vi "Main.vi"() -> ()   [LabVIEW 2013]
uses:
  Ctl/States.ctl
  Ctl/Setup.ctl
  GlobValue.vi
panel:
  out "SN_Head":string
  out "SN_Length":i32
  out "error out":errorcluster caption="错误输出"
  in  "IdentifyReady":bool
  in  "SlotReady":bool
  out "直通率":string
  out "Failed":u32
  out "Tested":u32
  out "Passed":u32
  in  "Next":bool
  out "测试失败项目":string
  in  "Starttime":u32
  out "Pass Yeild":dbl(graph)
  in  "GUIRef":T1
  in  "Start":bool
  in  "测试模式":u16(ring) items=["生产模式", "调试模式", "循环模式", "停止测试"]
  in  "循环次数":u32
  in  "产品标识":string
  out "测试结果":bool
  out "TBOX状态":bool
  in  "CheckOut":bool
  in  "Clear":bool
  out "进度条":i32(slide) scale=0.0..100.0
  out "测试时间":dbl
  out "分类测试结果":T2
  in  "中止":bool
  in  "Setup":bool
  out "运行Log":string
  in  "测试结果栏":i32(listbox)
  out "测试状态":string
  in  "Return":bool
  in  "产品名称":string
  in  "产品型号":u16(ring) items=["1802", "1805", "1831"]
  # "休眠唤醒测试"
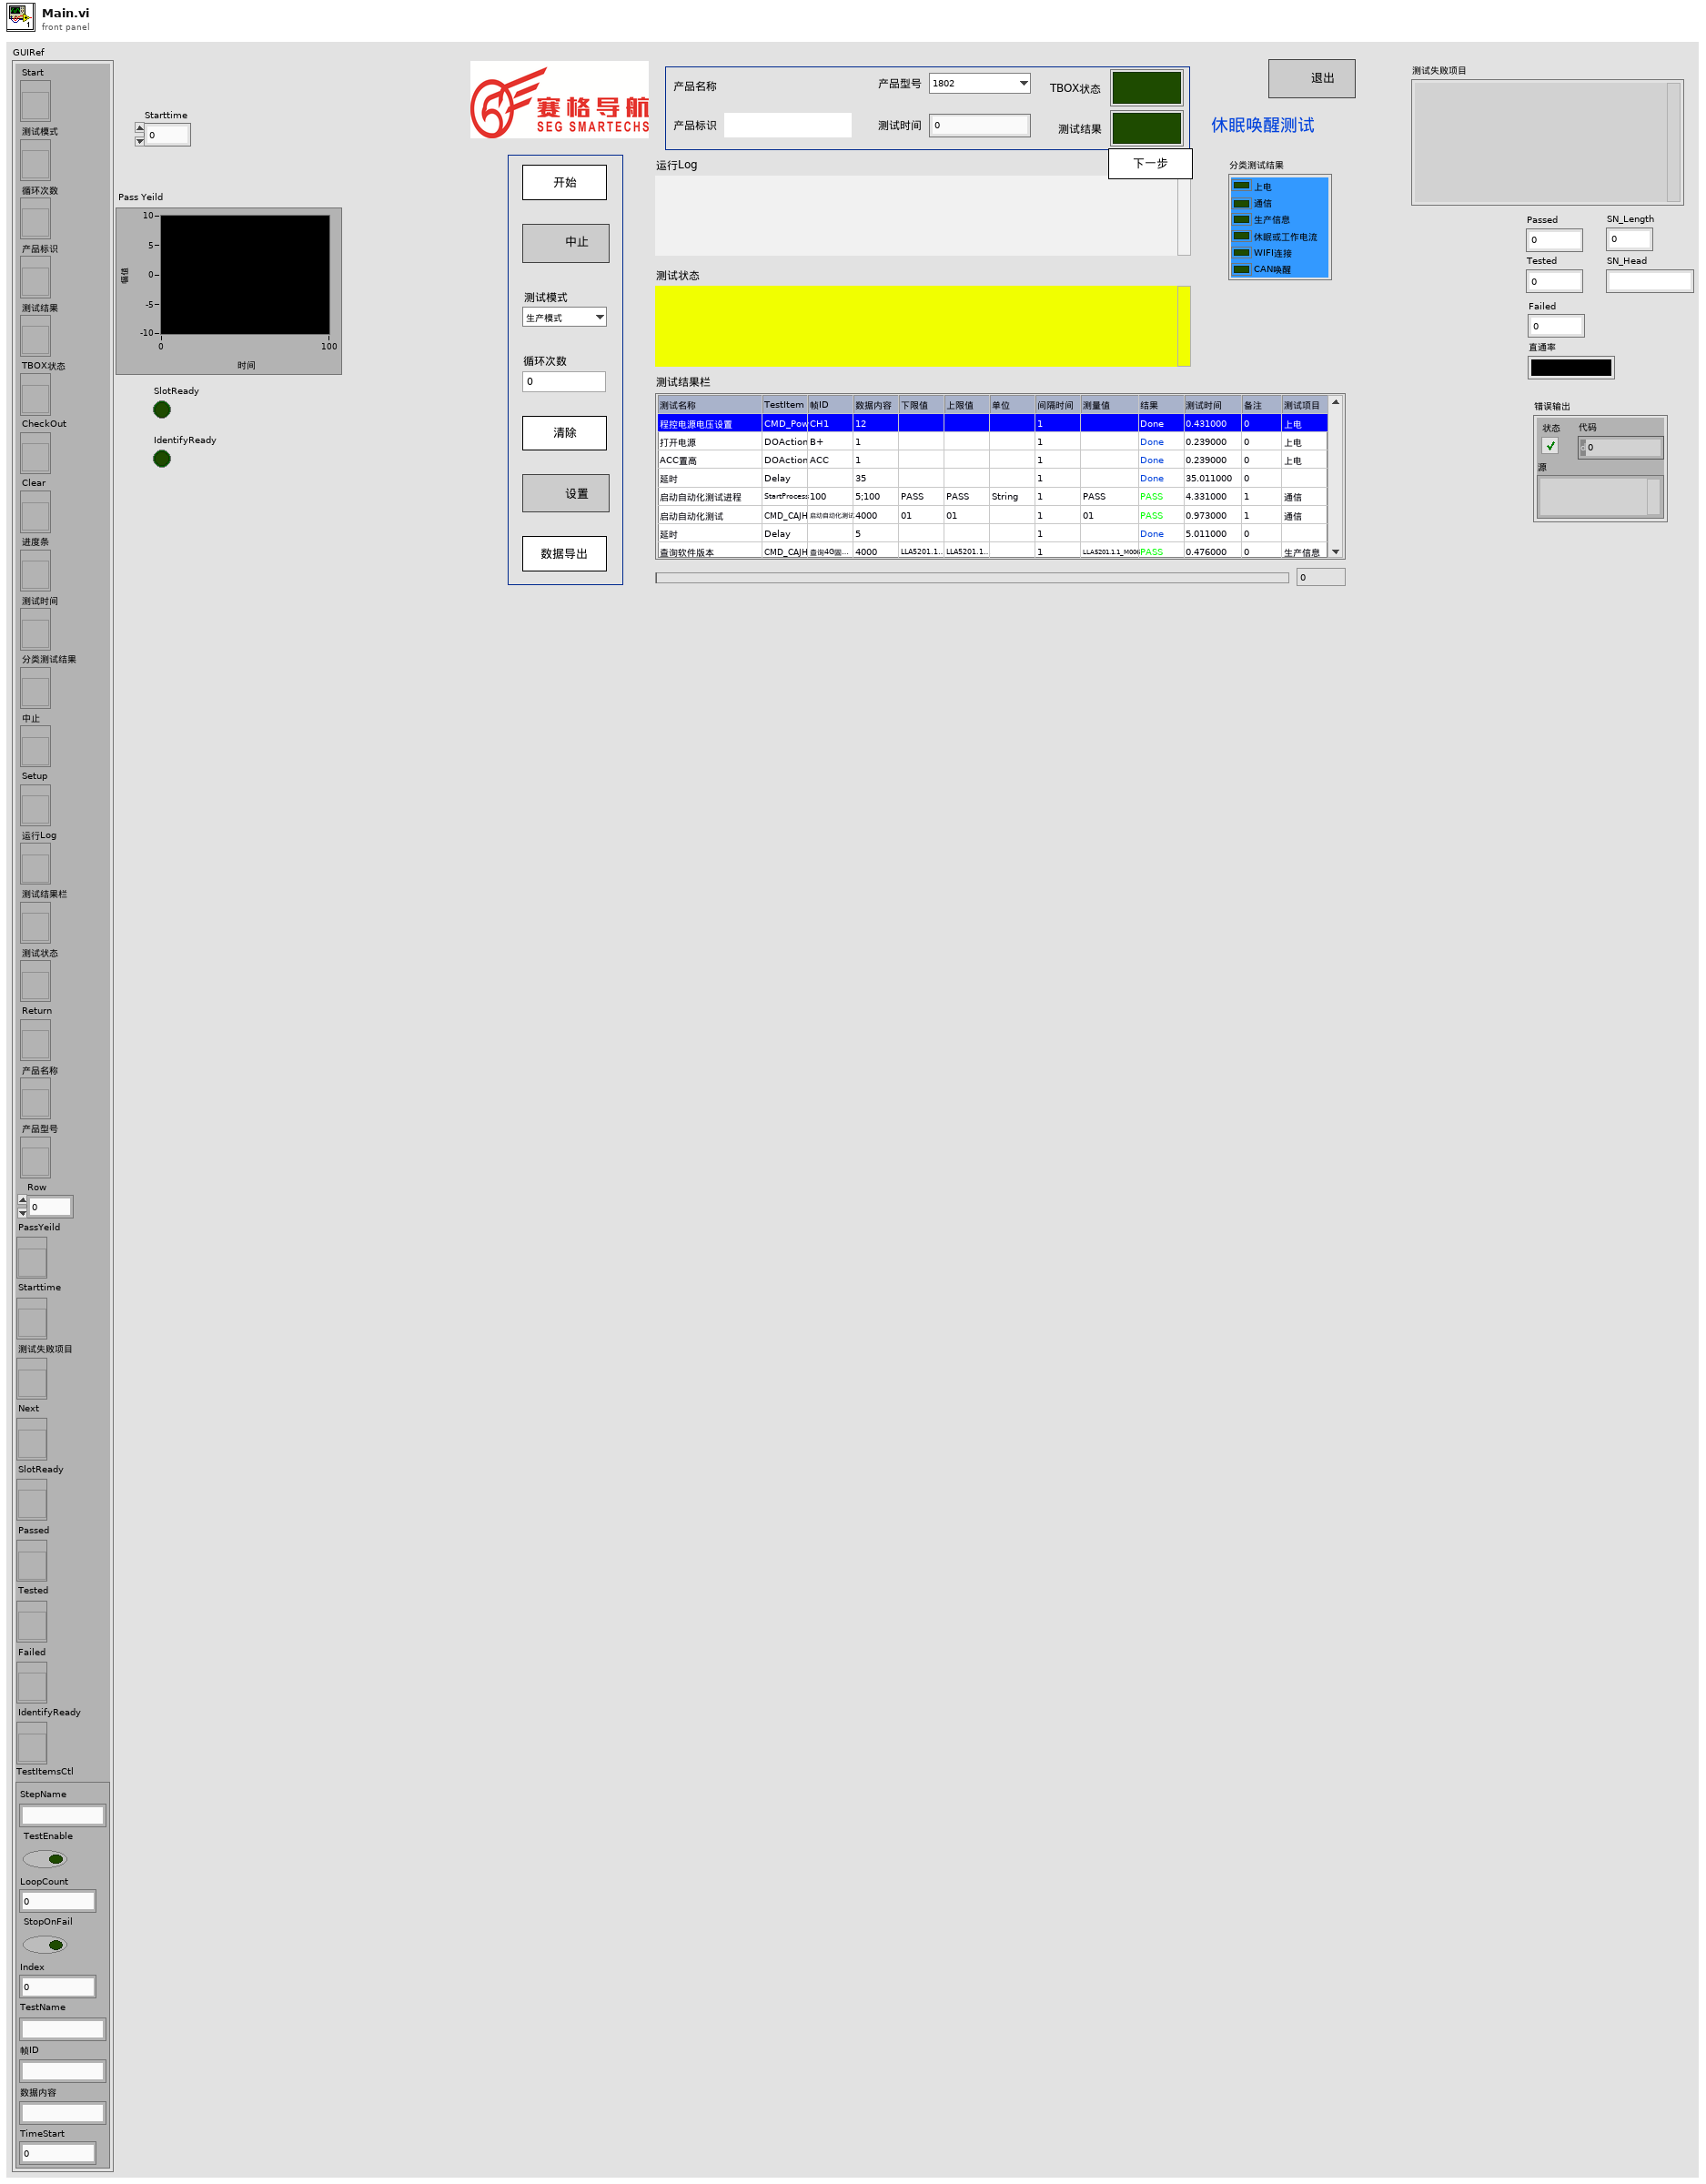
[diagram p1: front panel]
types:
  T1 = typedef "控件.ctl" = cluster{"Start":refnum<vi>, "测试模式":refnum<vi>, "循环次数":refnum<vi>, "产品标识":refnum<vi>, "测试结果":refnum<vi>, "TBOX状态":refnum<vi>, "CheckOut":refnum<vi>, "Clear":refnum<vi>, "进度条":refnum<vi>, "测试时间":refnum<vi>, "分类测试结果":refnum<vi>, "中止":refnum<vi>, "Setup":refnum<vi>, "运行Log":refnum<vi>, "测试结果栏":refnum<vi>, "测试状态":refnum<vi>, "Return":refnum<vi>, "产品名称":refnum<vi>, "产品型号":refnum<vi>, "Row":i32, "PassYeild":refnum<vi>, "Starttime":refnum<vi>, "测试失败项目":refnum<vi>, "Next":refnum<vi>, "SlotReady":refnum<vi>, "Passed":refnum<vi>, "Tested":refnum<vi>, "Failed":refnum<vi>, "IdentifyReady":refnum<vi>, "TestItemsCtl":cluster{"StepName":string, "TestEnable":bool, "LoopCount":u32, "StopOnFail":bool, "Index":u32, "TestName":string, "帧ID":string, "数据内容":string, "TimeStart":u32}}
  T2 = cluster{"电流":bool, "SD卡":bool, "USB":bool, "收音机":bool, "DVD":bool, "蓝牙":bool, "IPOD":bool, "终端":bool, "数字电视":bool, "AuxIn":bool, "按键":bool, "ILL检测":bool, "刹车检测":bool, "倒车检测":bool, "方控":bool, "导航":bool, "USB1":bool}
  T3 = enum8{"Enabled", "Disabled", "Disabled and Grayed Out"}
  T4 = typedef "States.ctl" = enum16{"Init", "PreUUT", "Idle", "SetUp", "TestSequence", "PostUUT", "StopTest", "Debug Mode", "Selection Mode", "Loop Mode", "Error", "Wait"}
  T5 = typedef "Setup.ctl" = cluster{"TestedNum":u32, "PassedNum":u32, "FailedNum":u32, "Slot1TestedNum":u32, "Slot2TestedNum":u32, "Slot3TestedNum":u32, "Slot4TestedNum":u32, "GuiVer":string, "LimitFileVer":string, "Login Name":string, "Password":string, "SN_Head":string, "SN_Length":i32, "AbortOnFail":bool, "DataBaseEnable?":bool, "FixtureID":string, "ShowSkipStep?":bool}
  T6 = enum32{"invalid app kind", "Development System", "Run Time System", "Student Edition", "Embedded LabVIEW", "Evaluation", "Custom"}
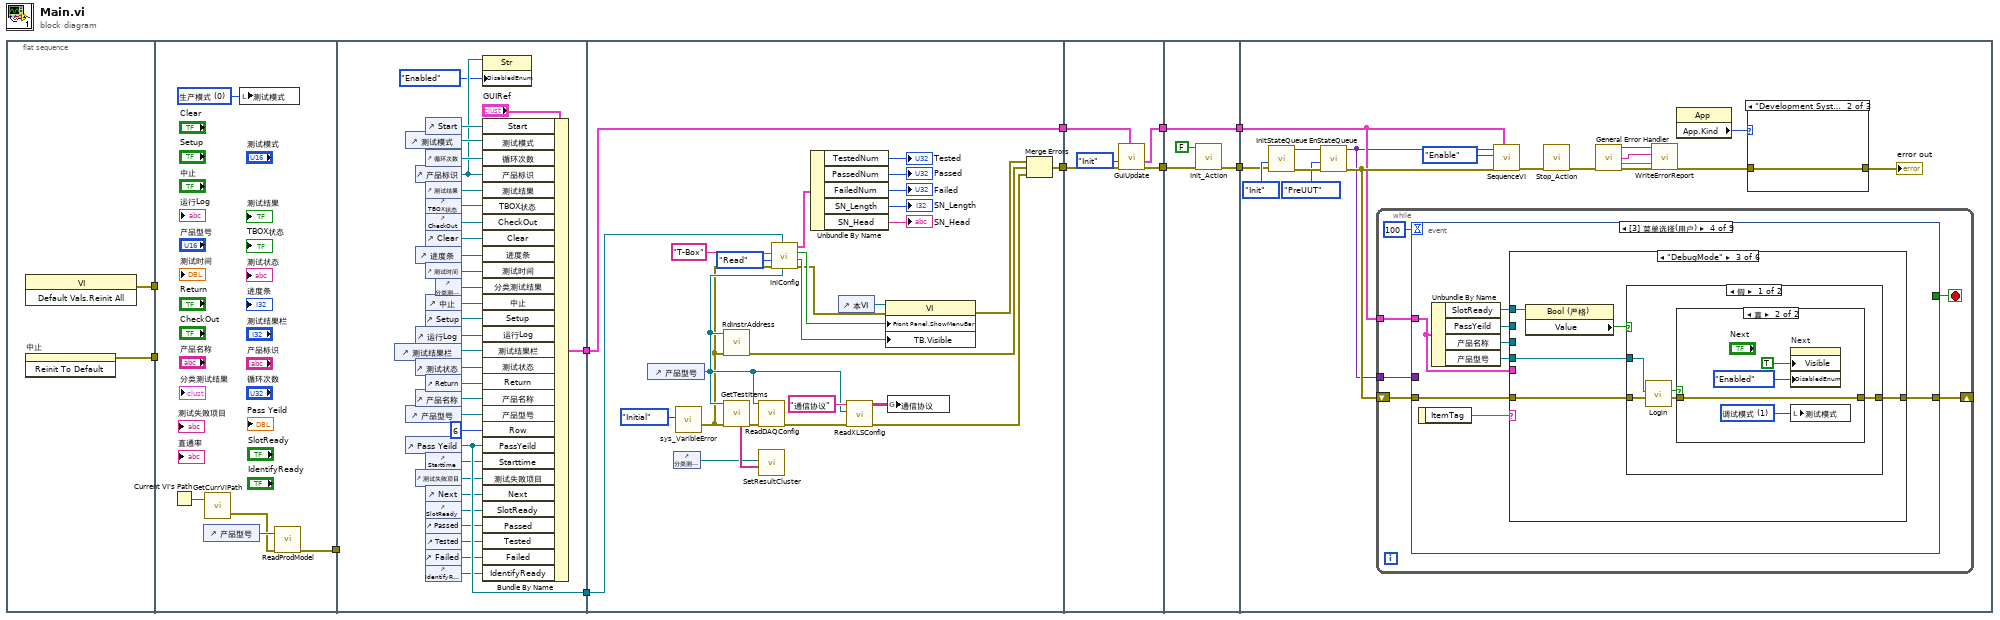
[diagram p0: block diagram]
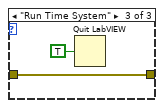
[diagram p3: hidden frame]
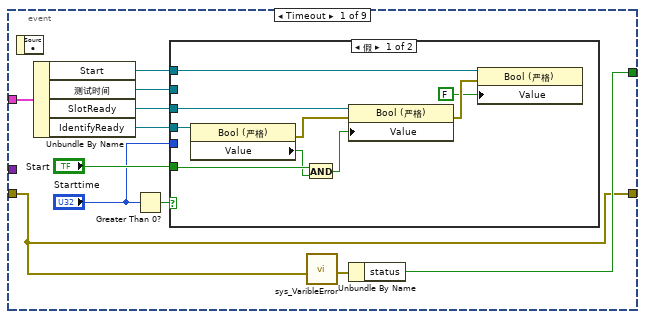
[diagram p4: hidden frame]
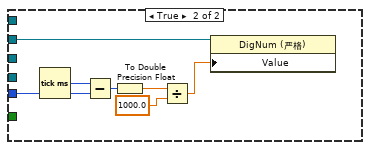
[diagram p5: hidden frame]
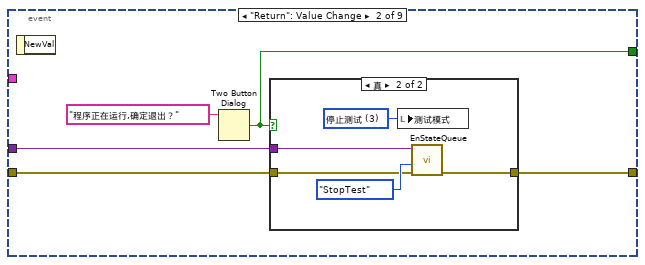
[diagram p6: hidden frame]
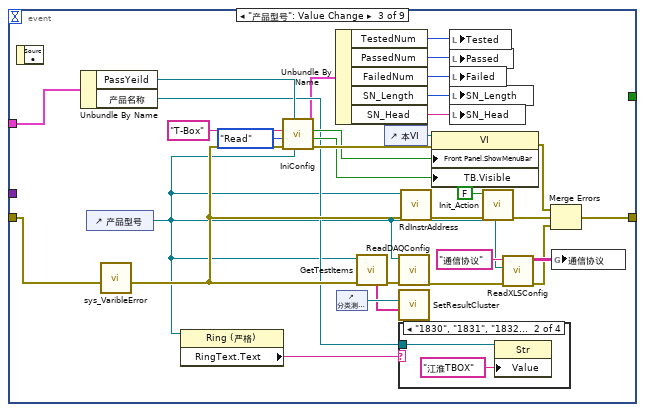
[diagram p8: hidden frame]
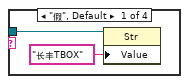
[diagram p9: hidden frame]
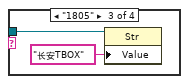
[diagram p10: hidden frame]
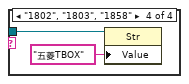
[diagram p11: hidden frame]
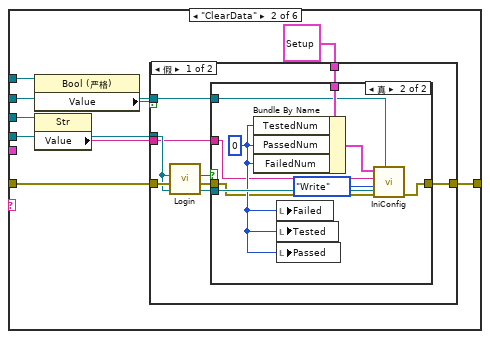
[diagram p13: hidden frame]
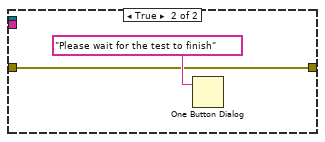
[diagram p15: hidden frame]
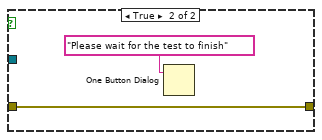
[diagram p17: hidden frame]
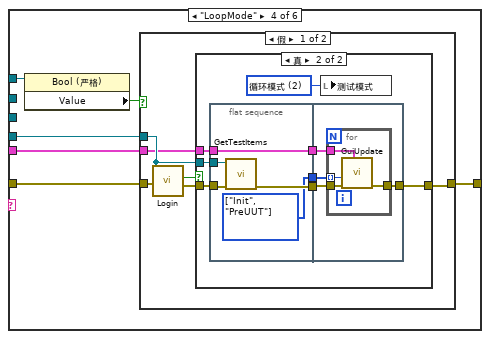
[diagram p18: hidden frame]
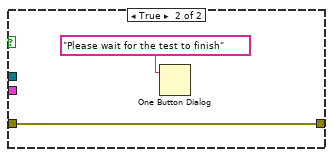
[diagram p20: hidden frame]
diagram:
  n1 = flat-sequence {
    tunnel: [w13] -> w11
    tunnel: [w12] -> w1
    tunnel: w11 -> [_]
    tunnel: [w15] -> w5
    tunnel: w1 -> [_]
    tunnel: [w31] -> w10
    tunnel: [w30] -> w9
    tunnel: w5 -> [_]
    tunnel: w10 -> [w57]
    tunnel: w9 -> [w63]
    tunnel: [w58] -> w8
    tunnel: [w57] -> w7
    tunnel: w8 -> [w82]
    tunnel: w7 -> [w79]
    tunnel: [w80] -> w6
    tunnel: [w78] -> w2
    tunnel: w6 -> [w86]
    tunnel: [w85] -> w4
    tunnel: [w84] -> w3
    tunnel: w2 -> [w84]
    tunnel: w4 -> [w102]
    tunnel: w3 -> [w88]
    frame #0 {
      n2 = invoke class="VI" method="Default Vals.Reinit All"() -> (error out=w13:errorcluster)  [unwired: 3 in, 2 out]
      n3 = invoke on="中止" class="Bool (严格)" method="Reinit To Default"() -> (error out=w12:errorcluster)  [unwired: 3 in, 2 out]
    }
    frame #1 {
      w17 = u16 0 items=["生产模式", "调试模式", "循环模式", "停止测试"] ("测试模式")
      n4 = Current VI's Path() -> (path=w18:path)
      n5 = control-ref of="产品型号"() -> (w16:refnum<vi>)
      n6 = call "GetCurrViPath.vi"("PathIn"=w18) -> ("error out"=w14:errorcluster)  [unwired: 1 in, 1 out]
      n7 = local write "测试模式"(w17) -> ()
      n8 = call "ReadProdModel.vi"("error in"=w14, "产品型号"=w16) -> ("error out"=w15:errorcluster)  [unwired: 9 in]
    }
    frame #2 {
      n9 = control-ref of="测试结果栏"() -> (w37:refnum<vi>)
      n10 = control-ref of="测试模式"() -> (w48:refnum<vi>)
      n11 = control-ref of="产品型号"() -> (w33:refnum<vi>)
      n12 = control-ref of="Pass Yeild"() -> (w30:refnum<vi>)
      n13 = control-ref of="产品标识"() -> (w20:refnum<vi>)
      n14 = control-ref of="进度条"() -> (w43:refnum<vi>)
      n15 = control-ref of="运行Log"() -> (w38:refnum<vi>)
      n16 = control-ref of="测试状态"() -> (w36:refnum<vi>)
      n17 = control-ref of="产品名称"() -> (w34:refnum<vi>)
      n18 = control-ref of="测试失败项目"() -> (w28:refnum<vi>)
      n19 = control-ref of="Start"() -> (w49:refnum<vi>)
      n20 = control-ref of="循环次数"() -> (w27:refnum<vi>)
      n21 = control-ref of="测试结果"() -> (w47:refnum<vi>)
      n22 = control-ref of="TBOX状态"() -> (w46:refnum<vi>)
      n23 = control-ref of="CheckOut"() -> (w45:refnum<vi>)
      n24 = control-ref of="Clear"() -> (w44:refnum<vi>)
      n25 = control-ref of="测试时间"() -> (w42:refnum<vi>)
      n26 = control-ref of="中止"() -> (w40:refnum<vi>)
      n27 = control-ref of="Setup"() -> (w39:refnum<vi>)
      n28 = control-ref of="Return"() -> (w35:refnum<vi>)
      n29 = control-ref of="Starttime"() -> (w29:refnum<vi>)
      n30 = control-ref of="Next"() -> (w25:refnum<vi>)
      n31 = control-ref of="SlotReady"() -> (w26:refnum<vi>)
      n32 = control-ref of="Passed"() -> (w24:refnum<vi>)
      n33 = control-ref of="Tested"() -> (w23:refnum<vi>)
      n34 = control-ref of="Failed"() -> (w22:refnum<vi>)
      n35 = control-ref of="IdentifyReady"() -> (w21:refnum<vi>)
      n36 = control-ref of="分类测试结果"() -> (w41:refnum<vi>)
      n37 = property class="Str"(reference=w20, "DisabledEnum"=T3."Enabled" ("禁用")) -> ()  [unwired: 1 in, 2 out]
      n38 = Bundle By Name(cluster="GUIRef", "Start"=w49, "测试模式"=w48, "循环次数"=w27, "产品标识"=w20, "测试结果"=w47, "TBOX状态"=w46, "CheckOut"=w45, "Clear"=w44, "进度条"=w43, "测试时间"=w42, "分类测试结果"=w41, "中止"=w40, "Setup"=w39, "运行Log"=w38, "测试结果栏"=w37, "测试状态"=w36, "Return"=w35, "产品名称"=w34, "产品型号"=w33, "Row"=6, "PassYeild"=w30, "Starttime"=w29, "测试失败项目"=w28, "Next"=w25, "SlotReady"=w26, "Passed"=w24, "Tested"=w23, "Failed"=w22, "IdentifyReady"=w21) -> (w31:T1)
    }
    frame #3 {
      n39 = control-ref of="产品型号"() -> (w70:refnum<vi>)
      n40 = control-ref of="分类测试结果"() -> (w71:refnum<vi>)
      n41 = call "sys_VaribleError.vi"("Operation"=enum16{"Initial", "Collect"}."Initial") -> ("ErrorOut"=w67:errorcluster)  [unwired: 10 in]
      n42 = call "RdInstrAddress.vi"("error in"=w67, "产品型号"=w70) -> ("error out"=w60:errorcluster)  [unwired: 8 in, 1 out]
      n43 = call "GetTestItems.vi"("error in"=w67, "产品型号"=w70) -> ("error out"=w76:errorcluster, "data"=w72:string[])  [unwired: 8 in]
      n44 = call "ReadDAQConfig.vi"("error in"=w76, "产品型号"=w70) -> ("error out"=w75:errorcluster)  [unwired: 8 in, 1 out]
      n45 = call "SetResultCluster.vi"("data"=w72, "测试结果簇"=w71) -> ()  [unwired: 10 in]
      n46 = call "IniConfig.vi"("产品型号"=w70, "PassYeild"=w63, "error in"=w67, "Operate"=enum16{"Write", "Read"}."Read", "ModelName"="T-Box") -> ("error out"=w62:errorcluster, "ShowToolBar"=w64:bool, "ShowMenu"=w65:bool, "ConfigOut"=w56:T5)  [unwired: 1 in, 2 out]
      n47 = Unbundle By Name(w56) -> ("TestedNum"=→"Tested":u32, "PassedNum"=→"Passed":u32, "FailedNum"=→"Failed":u32, "SN_Length"=→"SN_Length":i32, "SN_Head"=→"SN_Head":string)
      n48 = control-ref of="本VI"() -> (w66:refnum<vi>)
      n49 = call "ReadXLSConfig.vi"("error in"=w75, "产品型号"=w70, "XLSName"="通信协议") -> ("error out"=w59:errorcluster, "Data"=w73:string[][])  [unwired: 7 in]
      n50 = property class="VI"(reference=w66, error in=w62, "Front Panel.ShowMenuBar"=w65, "TB.Visible"=w64) -> (error out=w61:errorcluster)  [unwired: 1 out]
      n51 = global write "GlobValue.vi" "通信协议"(w73) -> ()
      n52 = Merge Errors(w61, w60, w59) -> (w58:errorcluster)
    }
    frame #4 {
      n53 = call "GuiUpdate.vi"("GuiRef"=w79, "error in"=w82, "States"=States."Init") -> ("error out"=w80:errorcluster, "GuiRefOut"=w78:T1)  [unwired: 6 in, 1 out]
    }
    frame #5 {
      n54 = call "Init_Action.vi"("error in"=w86, "AutoDetPort"=FALSE) -> ("error out"=w85:errorcluster)  [unwired: 9 in]
    }
    frame #6 {
      n55 = call "InitStateQueue.vi"("error in"=w102, "States"=States."Init") -> ("error out"=w101:errorcluster, "QueueOut"=w90:variant)  [unwired: 8 in]
      n56 = call "EnStateQueue.vi"("error in"=w101, "States"=States."PreUUT", "QueueIn"=w90) -> ("error out"=w89:errorcluster, "QueueOut"=w87:variant)  [unwired: 7 in]
      n57 = while {
        tunnel: w87 -> [w112]
        shift-right: [w109] -> _
        shift-left: w89 -> [w110]
        tunnel: w88 -> [w108]
        stop <- w111 stop-if-true
        n58 = event shown="[3] 菜单选择(用户)" {
          selector: _ -> [_ _ _ _ _ _ _ _ _]
          dyn-events: _ -> [_ _ _ _ _ _ _ _ _]
          timeout: 100 -> [_ _ _ _ _ _ _ _ _]
          tunnel: w112 -> [_ w144 _ _ w321 _ _ _ _]
          tunnel: [w116 w143 _ _ _ _ _ _ _] -> w111
          tunnel: w110 -> [w115 w142 w166 w194 w320 w330 w354 w392 w396]
          tunnel: [w115 w141 w167 w192 w319 w330 w353 w391 w394] -> w109
          tunnel: w108 -> [w122 _ w161 w191 _ w333 w356 w393 w400]
          event Timeout {
            n59 = event-data() -> ()  [unwired: 1 in, 1 out]
            n60 = Unbundle By Name(w122) -> ("Start"=w114:refnum<vi>, "测试时间"=w118:refnum<vi>, "SlotReady"=w120:refnum<vi>, "IdentifyReady"=w121:refnum<vi>)
            n61 = Greater Than 0?(x="Starttime") -> (x > 0?=w124:bool)
            n62 = case shown="假" w124 {
              tunnel: "Start" -> [w133 _]
              tunnel: w121 -> [w132 _]
              tunnel: w120 -> [w130 _]
              tunnel: "Starttime" -> [_ w139]
              tunnel: w118 -> [_ w134]
              tunnel: w114 -> [w127 _]
              frame False {
                n63 = property class="Bool (严格)"(reference=w132) -> (error out=w128:errorcluster, "Value"=w131:bool)  [unwired: 1 in, 1 out]
                n64 = And(x=w133, y=w131) -> (x .and. y?=w129:bool)
                n65 = property class="Bool (严格)"(reference=w130, error in=w128, "Value"=w129) -> (error out=w126:errorcluster)  [unwired: 1 out]
                n66 = property class="Bool (严格)"(reference=w127, error in=w126, "Value"=FALSE) -> ()  [unwired: 2 out]
              }
              frame True {
                n67 = Tick Count (ms)() -> (millisecond timer value=w140:u32)
                n68 = Subtract(x=w140, y=w139) -> (x-y=w138:u32)
                n69 = To Double Precision Float(number=w138) -> (double precision float=w137:dbl)
                n70 = Divide(x=w137, y=1000.0) -> (x/y=w135:dbl)
                n71 = property class="DigNum (严格)"(reference=w134, "Value"=w135) -> ()  [unwired: 1 in, 2 out]
              }
            }
            n72 = call "sys_VaribleError.vi"("ErrorIn"=w115) -> ("ErrorOut"=w117:errorcluster)  [unwired: 10 in]
            n73 = Unbundle By Name(w117) -> ("status"=w116:bool)
          }
          event "Return": Value Change {
            n74 = event-data() -> ()  [unwired: 1 in, 1 out]
            n75 = Two Button Dialog(message="程序正在运行,确定退出？" ("消息")) -> (T button?=w143:bool)  [unwired: 2 in]
            n76 = case shown="真" w143 {
              tunnel: w144 -> [_ w150]
              tunnel: w142 -> [w146 w148]
              tunnel: [w146 w147] -> w141
              frame False {
              }
              frame True {
                w151 = u16 3 items=["生产模式", "调试模式", "循环模式", "停止测试"] ("测试模式")
                n77 = local write "测试模式"(w151) -> ()
                n78 = call "EnStateQueue.vi"("error in"=w148, "States"=States."StopTest", "QueueIn"=w150) -> ("error out"=w147:errorcluster)  [unwired: 7 in, 1 out]
              }
            }
          }
          event "产品型号": Value Change {
            n79 = event-data() -> ()  [unwired: 1 in, 1 out]
            n80 = Unbundle By Name(w161) -> ("PassYeild"=w165:refnum<vi>, "产品名称"=w159:refnum<vi>)
            n81 = control-ref of="产品型号"() -> (w158:refnum<vi>)
            n82 = call "sys_VaribleError.vi"("ErrorIn"=w166) -> ("ErrorOut"=w178:errorcluster)  [unwired: 10 in]
            n83 = property class="Ring (严格)"(reference=w158) -> ("RingText.Text"=w160:string)  [unwired: 1 in, 2 out]
            n84 = call "IniConfig.vi"("产品型号"=w158, "PassYeild"=w165, "error in"=w178, "Operate"=enum16{"Write", "Read"}."Read", "ModelName"="T-Box") -> ("error out"=w182:errorcluster, "ShowToolBar"=w181:bool, "ShowMenu"=w180:bool, "ConfigOut"=w157:T5)  [unwired: 1 in, 2 out]
            n85 = Unbundle By Name(w157) -> ("TestedNum"=w156:u32, "PassedNum"=w155:u32, "FailedNum"=w154:u32, "SN_Length"=w153:i32, "SN_Head"=w152:string)
            n86 = control-ref of="分类测试结果"() -> (w175:refnum<vi>)
            n87 = call "GetTestItems.vi"("error in"=w178, "产品型号"=w158) -> ("error out"=w170:errorcluster, "data"=w174:string[])  [unwired: 8 in]
            n88 = control-ref of="本VI"() -> (w179:refnum<vi>)
            n89 = call "ReadDAQConfig.vi"("error in"=w170, "产品型号"=w158) -> ("error out"=w171:errorcluster)  [unwired: 8 in, 1 out]
            n90 = call "SetResultCluster.vi"("data"=w174, "测试结果簇"=w175) -> ()  [unwired: 10 in]
            n91 = case shown="\"1830\", \"1831\", \"1832\"" w160 {
              tunnel: w159 -> [w183 w186 w188 w190]
              frame "假", Default {
                n92 = property class="Str"(reference=w183, "Value"="长丰TBOX" ("值")) -> ()  [unwired: 1 in, 2 out]
              }
              frame "1830", "1831", "1832" {
                n93 = property class="Str"(reference=w186, "Value"="江淮TBOX" ("值")) -> ()  [unwired: 1 in, 2 out]
              }
              frame "1805" {
                n94 = property class="Str"(reference=w188, "Value"="长安TBOX" ("值")) -> ()  [unwired: 1 in, 2 out]
              }
              frame "1802", "1803", "1858" {
                n95 = property class="Str"(reference=w190, "Value"="五菱TBOX" ("值")) -> ()  [unwired: 1 in, 2 out]
              }
            }
            n96 = call "RdInstrAddress.vi"("error in"=w178, "产品型号"=w158) -> ("error out"=w163:errorcluster)  [unwired: 8 in, 1 out]
            n97 = property class="VI"(reference=w179, error in=w182, "Front Panel.ShowMenuBar"=w180, "TB.Visible"=w181) -> (error out=w169:errorcluster)  [unwired: 1 out]
            n98 = local write "Tested"(w156) -> ()
            n99 = local write "Passed"(w155) -> ()
            n100 = local write "Failed"(w154) -> ()
            n101 = local write "SN_Length"(w153) -> ()
            n102 = local write "SN_Head"(w152) -> ()
            n103 = call "Init_Action.vi"("error in"=w163, "AutoDetPort"=FALSE) -> ("error out"=w162:errorcluster)  [unwired: 9 in]
            n104 = call "ReadXLSConfig.vi"("error in"=w171, "产品型号"=w158, "XLSName"="通信协议") -> ("error out"=w168:errorcluster, "Data"=w173:string[][])  [unwired: 7 in]
            n105 = Merge Errors(w169, w162, w168) -> (w167:errorcluster)
            n106 = global write "GlobValue.vi" "通信协议"(w173) -> ()
          }
          event Menu Selection (User) {
            n107 = event-data() -> ("ItemTag"=w198:string)  [unwired: 1 in]
            n108 = Unbundle By Name(w191) -> ("SlotReady"=w197:refnum<vi>, "PassYeild"=w193:refnum<vi>, "产品名称"=w195:refnum<vi>, "产品型号"=w196:refnum<vi>)
            n109 = case shown="\"DebugMode\"" w198 {
              tunnel: w197 -> [_ w208 w230 w251 w287 _]
              tunnel: w196 -> [_ w206 w232 w247 w283 w311]
              tunnel: w195 -> [_ w205 _ _ _ _]
              tunnel: w194 -> [w199 w204 w233 w248 w284 w315]
              tunnel: w193 -> [_ w202 _ _ _ _]
              tunnel: [w199 w200 w231 w249 w285 w312] -> w192
              tunnel: w191 -> [_ _ _ w246 w282 _]
              frame "", Default {
              }
              frame "ClearData" {
                n110 = property class="Bool (严格)"(reference=w208) -> ("Value"=w207:bool)  [unwired: 1 in, 2 out]
                n111 = property class="Str"(reference=w205) -> ("Value"=w201:string)  [unwired: 1 in, 2 out]
                n112 = case shown="假" w207 {
                  tunnel: w206 -> [w215 _]
                  tunnel: w204 -> [w216 w227]
                  tunnel: T5 {"TestedNum"=10, "PassedNum"=5, "FailedNum"=5, "Slot1TestedNum"=10, "Slot2TestedNum"=10, "Slot3TestedNum"=10, "Slot4TestedNum"=10, "GuiVer"="1.0", "LimitFileVer"="1.0", "Login Name"="", "Password"="", "SN_Head"="0", "SN_Length"=1, "AbortOnFail"=FALSE, "DataBaseEnable?"=FALSE, "FixtureID"="", "ShowSkipStep?"=FALSE} ("ConfigOut") -> [w213 _]
                  tunnel: w202 -> [w212 _]
                  tunnel: w201 -> [w211 _]
                  tunnel: [w209 w227] -> w200
                  frame False {
                    n113 = call "Login.vi"("error in"=w216, "产品型号"=w215) -> ("error out"=w210:errorcluster, "Access"=w214:bool)  [unwired: 8 in]
                    n114 = case shown="真" w214 {
                      tunnel: w215 -> [_ w226]
                      tunnel: w213 -> [_ w225]
                      tunnel: w212 -> [_ w221]
                      tunnel: w211 -> [_ w220]
                      tunnel: w210 -> [w217 w219]
                      tunnel: [w217 w218] -> w209
                      frame False {
                      }
                      frame True {
                        w223 = u32 0
                        n115 = Bundle By Name(cluster=w225, "TestedNum"=w223, "PassedNum"=w223, "FailedNum"=w223) -> (w224:T5)
                        n116 = local write "Failed"(w223) -> ()
                        n117 = local write "Tested"(w223) -> ()
                        n118 = local write "Passed"(w223) -> ()
                        n119 = call "IniConfig.vi"("产品型号"=w226, "PassYeild"=w221, "error in"=w219, "Operate"=enum16{"Write", "Read"}."Write", "ModelName"=w220, "ConfigIn"=w224) -> ("error out"=w218:errorcluster)  [unwired: 5 out]
                      }
                    }
                  }
                  frame True {
                    n120 = One Button Dialog(message="Please wait for the test to finish" ("消息")) -> ()  [unwired: 1 in, 1 out]
                  }
                }
              }
              frame "DebugMode" {
                n121 = property class="Bool (严格)"(reference=w230) -> ("Value"=w229:bool)  [unwired: 1 in, 2 out]
                n122 = case shown="假" w229 {
                  tunnel: w233 -> [w238 w245]
                  tunnel: w232 -> [w237 _]
                  tunnel: [w234 w245] -> w231
                  frame False {
                    n123 = call "Login.vi"("error in"=w238, "产品型号"=w237) -> ("error out"=w235:errorcluster, "Access"=w236:bool)  [unwired: 8 in]
                    n124 = case shown="真" w236 {
                      tunnel: w235 -> [w239 w240]
                      tunnel: [w239 w240] -> w234
                      frame False {
                      }
                      frame True {
                        w243 = u16 1 items=["生产模式", "调试模式", "循环模式", "停止测试"] ("测试模式")
                        n125 = property on="Next" class="Bool (严格)"("Visible"=TRUE ("可见"), "DisabledEnum"=T3."Enabled" ("禁用")) -> ()  [unwired: 2 in, 2 out]
                        n126 = local write "测试模式"(w243) -> ()
                      }
                    }
                  }
                  frame True {
                    n127 = One Button Dialog(message="Please wait for the test to finish" ("消息")) -> ()  [unwired: 1 in, 1 out]
                  }
                }
              }
              frame "LoopMode" {
                n128 = property class="Bool (严格)"(reference=w251) -> ("Value"=w250:bool)  [unwired: 1 in, 2 out]
                n129 = case shown="假" w250 {
                  tunnel: [w253 w281] -> w249
                  tunnel: w248 -> [w257 w281]
                  tunnel: w247 -> [w254 _]
                  tunnel: w246 -> [w252 _]
                  frame False {
                    n130 = call "Login.vi"("error in"=w257, "产品型号"=w254) -> ("error out"=w255:errorcluster, "Access"=w256:bool)  [unwired: 8 in]
                    n131 = case shown="真" w256 {
                      tunnel: w255 -> [w258 w266]
                      tunnel: w254 -> [_ w265]
                      tunnel: [w258 w263] -> w253
                      tunnel: w252 -> [_ w260]
                      frame False {
                      }
                      frame True {
                        w259 = u16 2 items=["生产模式", "调试模式", "循环模式", "停止测试"] ("测试模式")
                        n132 = flat-sequence {
                          tunnel: w266 -> [w271]
                          tunnel: w265 -> [w270]
                          tunnel: [w269] -> w264
                          tunnel: [w268] -> w262
                          tunnel: [w267] -> w261
                          tunnel: w260 -> [w267]
                          tunnel: w264 -> [w275]
                          tunnel: [w274] -> w263
                          tunnel: w262 -> [w273]
                          tunnel: w261 -> [w272]
                          frame #0 {
                            w268 = T4[] [enum."Init", enum."PreUUT"] items=["Init", "PreUUT", "Idle", "SetUp", "TestSequence", "PostUUT", "StopTest", "Debug Mode", "Selection Mode", "Loop Mode", "Error", "Wait"]
                            n133 = call "GetTestItems.vi"("error in"=w271, "产品型号"=w270) -> ("error out"=w269:errorcluster)  [unwired: 8 in, 1 out]
                          }
                          frame #1 {
                            n134 = for {
                              tunnel: w275 -> [w279]
                              tunnel: [w278] -> w274
                              tunnel: w273 -> [w277] mode=indexing
                              tunnel: w272 -> [w276]
                              n135 = call "GuiUpdate.vi"("GuiRef"=w276, "error in"=w279, "States"=w277) -> ("error out"=w278:errorcluster)  [unwired: 6 in, 2 out]
                            }
                          }
                        }
                        n136 = local write "测试模式"(w259) -> ()
                      }
                    }
                  }
                  frame True {
                    n137 = One Button Dialog(message="Please wait for the test to finish" ("消息")) -> ()  [unwired: 1 in, 1 out]
                  }
                }
              }
              frame "ProductionMode" {
                n138 = property class="Bool (严格)"(reference=w287) -> ("Value"=w286:bool)  [unwired: 1 in, 2 out]
                n139 = case shown="假" w286 {
                  tunnel: [w294 w310] -> w285
                  tunnel: w284 -> [w288 w310]
                  tunnel: w283 -> [w295 _]
                  tunnel: w282 -> [w293 _]
                  frame False {
                    w289 = u16 0 items=["生产模式", "调试模式", "循环模式", "停止测试"] ("测试模式")
                    n140 = flat-sequence {
                      tunnel: w288 -> [w300]
                      tunnel: w295 -> [w299]
                      tunnel: [w298] -> w292
                      tunnel: [w297] -> w291
                      tunnel: [w296] -> w290
                      tunnel: w293 -> [w296]
                      tunnel: w292 -> [w304]
                      tunnel: [w303] -> w294
                      tunnel: w291 -> [w302]
                      tunnel: w290 -> [w301]
                      frame #0 {
                        w297 = T4[] [enum."Init", enum."PreUUT"] items=["Init", "PreUUT", "Idle", "SetUp", "TestSequence", "PostUUT", "StopTest", "Debug Mode", "Selection Mode", "Loop Mode", "Error", "Wait"]
                        n141 = call "GetTestItems.vi"("error in"=w300, "产品型号"=w299) -> ("error out"=w298:errorcluster)  [unwired: 8 in, 1 out]
                      }
                      frame #1 {
                        n142 = for {
                          tunnel: w304 -> [w308]
                          tunnel: [w307] -> w303
                          tunnel: w302 -> [w306] mode=indexing
                          tunnel: w301 -> [w305]
                          n143 = call "GuiUpdate.vi"("GuiRef"=w305, "error in"=w308, "States"=w306) -> ("error out"=w307:errorcluster)  [unwired: 6 in, 2 out]
                        }
                      }
                    }
                    n144 = local write "测试模式"(w289) -> ()
                  }
                  frame True {
                    n145 = One Button Dialog(message="Please wait for the test to finish" ("消息")) -> ()  [unwired: 1 in, 1 out]
                  }
                }
              }
              frame "User" {
                n146 = call "Login.vi"("error in"=w315, "产品型号"=w311) -> ("error out"=w313:errorcluster, "Access"=w314:bool)  [unwired: 8 in]
                n147 = case shown="真" w314 {
                  tunnel: w313 -> [w316 w318]
                  tunnel: [w316 w318] -> w312
                  tunnel: w311 -> [_ w317]
                  frame False {
                  }
                  frame True {
                    n148 = call "ModifyUser.vi"("产品型号"=w317) -> ()  [unwired: 11 in]
                  }
                }
              }
            }
          }
          event Panel Close? {
            n149 = event-data() -> ()  [unwired: 1 in, 1 out]
            n150 = Two Button Dialog(message="程序正在运行,确定退出？" ("消息")) -> (T button?=w322:bool)  [unwired: 2 in]
            n151 = case shown="真" w322 {
              tunnel: w321 -> [_ w328]
              tunnel: w320 -> [w324 w326]
              tunnel: [w324 w325] -> w319
              frame False {
              }
              frame True {
                w329 = u16 3 items=["生产模式", "调试模式", "循环模式", "停止测试"] ("测试模式")
                n152 = local write "测试模式"(w329) -> ()
                n153 = call "EnStateQueue.vi"("error in"=w326, "States"=States."StopTest", "QueueIn"=w328) -> ("error out"=w325:errorcluster)  [unwired: 7 in, 1 out]
              }
            }
            n154 = event-data("Discard?"=w322) -> ()  [unwired: 1 in, 1 out]
          }
          event "产品标识": Value Change {
            n155 = event-data() -> ("CtlRef"=w342:refnum<vi>, "NewVal"=w344:string)  [unwired: 1 in]
            n156 = Unbundle By Name(w333) -> ("产品标识"=w331:refnum<vi>, "IdentifyReady"=w332:refnum<vi>)
            n157 = local read "SN_Head"() -> (w338:string)
            n158 = To Upper Case(1:w344) -> (0:w343:string)
            n159 = call <vilib>:"Trim Whitespace.vi"("string"=w343) -> ("trimmed string"=w339:string)  [unwired: 1 in]
            n160 = Match Pattern(string=w339, regular expression=w338) -> (offset past match=w337:i32)  [unwired: 1 in, 3 out]
            n161 = local read "SN_Length"() -> (w340:i32)
            n162 = property class="Str"(reference=w342, "Value"=w339) -> ()  [unwired: 1 in, 2 out]
            n163 = Greater Or Equal To 0?(x=w337) -> (x >= 0?=w335:bool)
            n164 = String Length(string=w339) -> (length=w341:i32)
            n165 = Equal?(x=w341, y=w340) -> (x = y?=w336:bool)
            n166 = Compound Arithmetic op=AND(w336, w335) -> (w334:bool)
            n167 = case shown="真" w334 {
              tunnel: w332 -> [_ w352]
              tunnel: w331 -> [w347 _]
              frame False {
                n168 = flat-sequence {
                  tunnel: [w349] -> w348
                  tunnel: w347 -> [w349]
                  frame #0 {
                    n169 = One Button Dialog(message="产品标识输入\n错误，请检查！") -> ()  [unwired: 1 in, 1 out]
                  }
                }
                n170 = property class="Str"(reference=w348, "Key Focus"=TRUE ("键选中"), "Value"="") -> ()  [unwired: 1 in, 2 out]
              }
              frame True {
                n171 = property class="Bool (严格)"(reference=w352, "Value"=TRUE ("值")) -> ()  [unwired: 1 in, 2 out]
              }
            }
          }
          event "Clear": Value Change {
            n172 = event-data() -> ("NewVal"=w355:bool)  [unwired: 1 in]
            n173 = case shown="真" w355 {
              tunnel: w356 -> [_ w365]
              tunnel: w354 -> [w357 w359]
              tunnel: [w357 w358] -> w353
              frame False {
              }
              frame True {
                n174 = Unbundle By Name(w365) -> ("SlotReady"=w367:refnum<vi>)
                n175 = Unbundle By Name(w365) -> ("产品型号"=w360:refnum<vi>, "PassYeild"=w361:refnum<vi>, "产品名称"=w363:refnum<vi>)
                n176 = property class="Bool (严格)"(reference=w367) -> ("Value"=w366:bool)  [unwired: 1 in, 2 out]
                n177 = property class="Str"(reference=w363) -> ("Value"=w362:string)  [unwired: 1 in, 2 out]
                n178 = case shown="真" w366 {
                  tunnel: T5 {"TestedNum"=10, "PassedNum"=5, "FailedNum"=5, "Slot1TestedNum"=10, "Slot2TestedNum"=10, "Slot3TestedNum"=10, "Slot4TestedNum"=10, "GuiVer"="1.0", "LimitFileVer"="1.0", "Login Name"="", "Password"="", "SN_Head"="0", "SN_Length"=1, "AbortOnFail"=FALSE, "DataBaseEnable?"=FALSE, "FixtureID"="", "ShowSkipStep?"=FALSE} ("ConfigOut") -> [w376 _]
                  tunnel: w362 -> [w375 _]
                  tunnel: w360 -> [w373 _]
                  tunnel: w361 -> [w374 _]
                  tunnel: w360 -> [w372 _]
                  tunnel: w359 -> [w369 w388]
                  tunnel: [w368 w388] -> w358
                  frame False {
                    n179 = call "Login.vi"("error in"=w369, "产品型号"=w372) -> ("error out"=w370:errorcluster, "Access"=w371:bool)  [unwired: 8 in]
                    n180 = case shown="真" w371 {
                      tunnel: w376 -> [_ w387]
                      tunnel: w375 -> [_ w385]
                      tunnel: w374 -> [_ w383]
                      tunnel: w373 -> [_ w382]
                      tunnel: w370 -> [w378 w380]
                      tunnel: [w378 w379] -> w368
                      frame False {
                        n181 = One Button Dialog(message="用户名或密码输入错误！" ("消息")) -> ()  [unwired: 1 in, 1 out]
                      }
                      frame True {
                        w381 = 0
                        n182 = Bundle By Name(cluster=w387, "TestedNum"=w381, "PassedNum"=w381, "FailedNum"=w381) -> (w386:T5)
                        n183 = local write "Failed"(w381) -> ()
                        n184 = local write "Tested"(w381) -> ()
                        n185 = local write "Passed"(w381) -> ()
                        n186 = call "IniConfig.vi"("产品型号"=w382, "PassYeild"=w383, "error in"=w380, "Operate"=enum16{"Write", "Read"}."Write", "ModelName"=w385, "ConfigIn"=w386) -> ("error out"=w379:errorcluster)  [unwired: 5 out]
                      }
                    }
                  }
                  frame True {
                    n187 = One Button Dialog(message="请等待测试结束后操作" ("消息")) -> ()  [unwired: 1 in, 1 out]
                  }
                }
              }
            }
          }
          event "中止": Value Change {
            n188 = event-data() -> ()  [unwired: 1 in, 1 out]
            n189 = call "GuiUpdate.vi"("GuiRef"=w393, "error in"=w392, "States"=States."StopTest") -> ("error out"=w391:errorcluster)  [unwired: 6 in, 2 out]
          }
          event "测试模式": Value Change {
            n190 = event-data() -> ("CtlRef"=w401:refnum<vi>)  [unwired: 1 in]
            n191 = Unbundle By Name(w400) -> ("循环次数"=w399:refnum<vi>)
            n192 = property class="Ring (严格)"(reference=w401, error in=w396) -> (error out=w395:errorcluster, "RingText.Text"=w402:string)  [unwired: 1 out]
            n193 = case shown="\"调试模式\", \"循环模式\"" w402 {
              tunnel: [T3."Enabled" ("禁用") T3."Disabled and Grayed Out" ("禁用")] -> w398
              frame "调试模式", "循环模式" {
              }
              frame "生产模式", Default {
              }
            }
            n194 = property class="DigNum (严格)"(reference=w399, error in=w395, "DisabledEnum"=w398, "Value"=u32 1 ("值")) -> (error out=w394:errorcluster)  [unwired: 1 out]
          }
        }
      }
      n195 = call "SequenceVI.vi"("GUIRefArray"=w88, "error in"=w89, "SlotEnable"=enum16{"Enable", "Disable"}."Enable", "QueueIn"=w87) -> ("error out"=w98:errorcluster)  [unwired: 7 in]
      n196 = call "Stop_Action.vi"("error in"=w98) -> ("error out"=w97:errorcluster)  [unwired: 10 in]
      n197 = call <vilib>:"General Error Handler.vi"("error in (no error)"=w97) -> ("error?"=w96:bool, "source out"=w95:string, "message"=w94:string, "error out"=w92:errorcluster)  [unwired: 10 in, 1 out]
      n198 = call "WriteErrorReport.vi"("message"=w94, "source out"=w95, "Error"=w96) -> ()  [unwired: 9 in]
      n199 = property class="App"() -> ("App.Kind"=w93:T6)  [unwired: 2 in, 2 out]
      n200 = case shown="\"Development System\"" w93 {
        tunnel: w92 -> [w104 w105 w106]
        tunnel: [w104 w105 w106] -> w91
        frame "invalid app kind", Default {
        }
        frame "Development System" {
        }
        frame "Run Time System" {
          n201 = Quit LabVIEW(quit? (T)=TRUE ("退出？(T)")) -> ()
        }
      }
      "error out" <- w91
    }
  }
